vi "centroid detection loop.vi"(7 "CCDs":string[](array[string]), 8 "error in (no error)":errorcluster, 9 "active cams":string[](array[string]), 10 "Detection in":T6 {"detection para"."Particle filtering"."Measurement Parameter" items=["Center of Mass X", "Center of Mass Y", "First Pixel X", "First Pixel Y", "Bounding Rect Left", "Bounding Rect Top", "Bounding Rect Right", "Bounding Rect Bottom", "Max Feret Diameter Start X", "Max Feret Diameter Start Y", "Max Feret Diameter End X", "Max Feret Diameter End Y", "Max Horiz. Segment Length Left", "Max Horiz. Segment Length Right", "Max Horiz. Segment Length Row", "-", "Bounding Rect Width", "Bounding Rect Height", "Bounding Rect Diagonal", "Perimeter", "Convex Hull Perimeter", "Holes' Perimeter", "Max Feret Diameter", "Equivalent Ellipse Major Axis", "Equivalent Ellipse Minor Axis", "Equivalent Ellipse Minor Axis (Feret)", "Equivalent Rect Long Side", "Equivalent Rect Short Side", "Equivalent Rect Diagonal", "Equivalent Rect Short Side (Feret)", "Average Horiz. Segment Length", "Average Vert. Segment Length", "Hydraulic Radius", "Waddel Disk Diameter", "-", "Area", "Holes' Area", "Particle & Holes' Area", "Convex Hull Area", "Image Area", "-", "Number of Holes", "Number of Horiz. Segments", "Number of Vert. Segments", "-", "Orientation", "Max Feret Diameter Orientation", "-", "% Area/Image Area", "% Area/(Particle & Holes' Area)", "Ratio of Equivalent Ellipse Axes", "Ratio of Equivalent Rect Sides", "-", "Elongation Factor", "Compactness Factor", "Heywood Circularity Factor", "Type Factor", "-", "Sum X", "Sum Y", "Sum XX", "Sum XY", "Sum YY", "Sum XXX", "Sum XXY", "Sum XYY", "Sum YYY", "-", "Moment of Inertia XX", "Moment of Inertia XY", "Moment of Inertia YY", "Moment of Inertia XXX", "Moment of Inertia XXY", "Moment of Inertia XYY", "Moment of Inertia YYY", "Norm. Moment of Inertia XX", "Norm. Moment of Inertia XY", "Norm. Moment of Inertia YY", "Norm. Moment of Inertia XXX", "Norm. Moment of Inertia XXY", "Norm. Moment of Inertia XYY", "Norm. Moment of Inertia YYY", "Hu Moment 1", "Hu Moment 2", "Hu Moment 3", "Hu Moment 4", "Hu Moment 5", "Hu Moment 6", "Hu Moment 7"]; "detection para"."Particle filtering"."Range Lower Value" format="%.2f"; "detection para"."Particle filtering"."Range Upper Value" format="%.2f"; "detection para"."detection method" items=["clustering", "entropy", "metric", "moments", "inter-class variance"]; "detection para"."Filter" items=["No Filter", "Median Filter", "Low Pass Filter"]}, 11 "autodetect":bool) -> (0 "error out":errorcluster, 1 "# where centr y is 0":i32[](array[numeric]), 2 "Detection out":T5 {"detection para"."Particle filtering"."Measurement Parameter" items=["Center of Mass X", "Center of Mass Y", "First Pixel X", "First Pixel Y", "Bounding Rect Left", "Bounding Rect Top", "Bounding Rect Right", "Bounding Rect Bottom", "Max Feret Diameter Start X", "Max Feret Diameter Start Y", "Max Feret Diameter End X", "Max Feret Diameter End Y", "Max Horiz. Segment Length Left", "Max Horiz. Segment Length Right", "Max Horiz. Segment Length Row", "-", "Bounding Rect Width", "Bounding Rect Height", "Bounding Rect Diagonal", "Perimeter", "Convex Hull Perimeter", "Holes' Perimeter", "Max Feret Diameter", "Equivalent Ellipse Major Axis", "Equivalent Ellipse Minor Axis", "Equivalent Ellipse Minor Axis (Feret)", "Equivalent Rect Long Side", "Equivalent Rect Short Side", "Equivalent Rect Diagonal", "Equivalent Rect Short Side (Feret)", "Average Horiz. Segment Length", "Average Vert. Segment Length", "Hydraulic Radius", "Waddel Disk Diameter", "-", "Area", "Holes' Area", "Particle & Holes' Area", "Convex Hull Area", "Image Area", "-", "Number of Holes", "Number of Horiz. Segments", "Number of Vert. Segments", "-", "Orientation", "Max Feret Diameter Orientation", "-", "% Area/Image Area", "% Area/(Particle & Holes' Area)", "Ratio of Equivalent Ellipse Axes", "Ratio of Equivalent Rect Sides", "-", "Elongation Factor", "Compactness Factor", "Heywood Circularity Factor", "Type Factor", "-", "Sum X", "Sum Y", "Sum XX", "Sum XY", "Sum YY", "Sum XXX", "Sum XXY", "Sum XYY", "Sum YYY", "-", "Moment of Inertia XX", "Moment of Inertia XY", "Moment of Inertia YY", "Moment of Inertia XXX", "Moment of Inertia XXY", "Moment of Inertia XYY", "Moment of Inertia YYY", "Norm. Moment of Inertia XX", "Norm. Moment of Inertia XY", "Norm. Moment of Inertia YY", "Norm. Moment of Inertia XXX", "Norm. Moment of Inertia XXY", "Norm. Moment of Inertia XYY", "Norm. Moment of Inertia YYY", "Hu Moment 1", "Hu Moment 2", "Hu Moment 3", "Hu Moment 4", "Hu Moment 5", "Hu Moment 6", "Hu Moment 7"]; "detection para"."Particle filtering"."Range Lower Value" format="%.2f"; "detection para"."Particle filtering"."Range Upper Value" format="%.2f"; "detection para"."detection method" items=["clustering", "entropy", "metric", "moments", "inter-class variance"]; "detection para"."Filter" items=["No Filter", "Median Filter", "Low Pass Filter"]}, 3 "bounding rectangle":T1(array[cluster]), 4 "detected array":bool[](array[boolean]), 5 "Particle Reports (Pixels)":T2(array[cluster]))   [LabVIEW 2020]
uses:
  Ctrs/Detection all.ctl
  Ctrs/beam detection.ctl
  <userlib>/_OpenG.lib/array/array.llb/Filter 1D Array with Scalar (String)__ogtk.vi
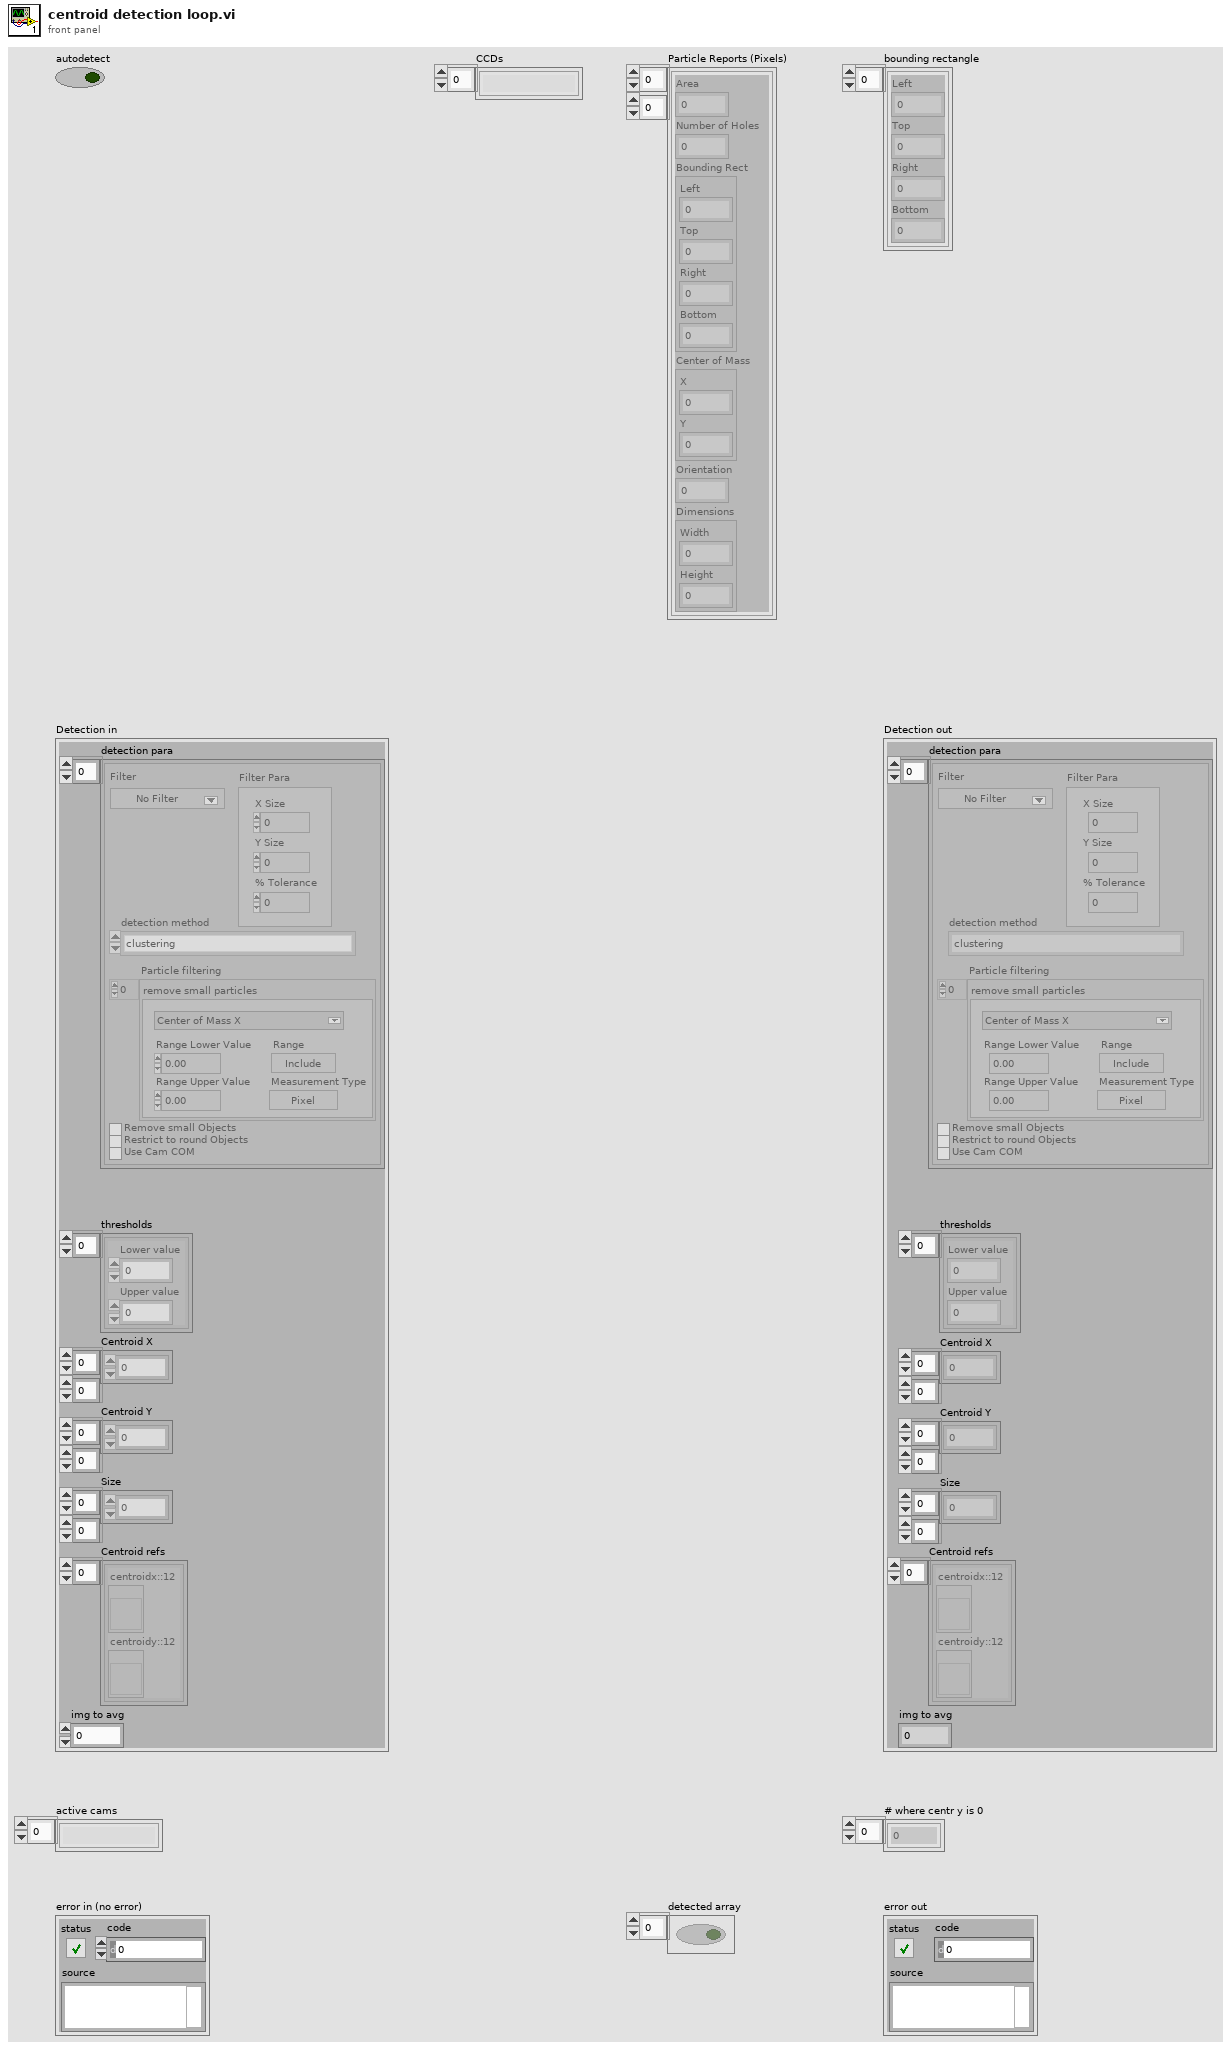
[diagram p1: front panel]
types:
  T1 = cluster{"Left":dbl, "Top":dbl, "Right":dbl, "Bottom":dbl}[]
  T2 = cluster{"Area":dbl, "Number of Holes":dbl, "Bounding Rect":cluster{"Left":dbl, "Top":dbl, "Right":dbl, "Bottom":dbl}, "Center of Mass":cluster{"X":dbl, "Y":dbl}, "Orientation":dbl, "Dimensions":cluster{"Width":dbl, "Height":dbl}}[][]
  T3 = typedef "beam detection.ctl" = cluster{"Filter":u16, "Filter Para":cluster{"X Size":i32, "Y Size":i32, "% Tolerance":i32}, "detection method":i32, "Particle filtering":cluster{"Measurement Parameter":T4, "Range Lower Value":dbl, "Range Upper Value":dbl, "Range":bool, "Measurement Type":bool}[], "Remove small Objects":bool, "Restrict to round Objects":bool, "Use Cam COM":bool}
  T4 = typedef "Particle Parameters" = i32
  T5 = cluster{"detection para":T3[], "thresholds":cluster{"Lower value":sgl, "Upper value":sgl}[], "Centroid X":dbl[][], "Centroid Y":dbl[][], "Size":dbl[][], "Centroid refs":cluster{"centroidx::12":refnum<vi>, "centroidy::12":refnum<vi>}[], "img to avg":i32}
  T6 = typedef "Detection all.ctl" = cluster{"detection para":T3[], "thresholds":cluster{"Lower value":sgl, "Upper value":sgl}[], "Centroid X":dbl[][], "Centroid Y":dbl[][], "Size":dbl[][], "Centroid refs":cluster{"centroidx::12":refnum<vi>, "centroidy::12":refnum<vi>}[], "img to avg":i32}
  T7 = cluster{"centroidx::12":refnum<vi>, "centroidy::12":refnum<vi>}[]
  T8 = cluster{"centroidx::12":refnum<vi>, "centroidy::12":refnum<vi>}
  T9 = cluster{"Left":dbl, "Top":dbl, "Right":dbl, "Bottom":dbl}
  T10 = cluster{"Area":dbl, "Number of Holes":dbl, "Bounding Rect":cluster{"Left":dbl, "Top":dbl, "Right":dbl, "Bottom":dbl}, "Center of Mass":cluster{"X":dbl, "Y":dbl}, "Orientation":dbl, "Dimensions":cluster{"Width":dbl, "Height":dbl}}[]
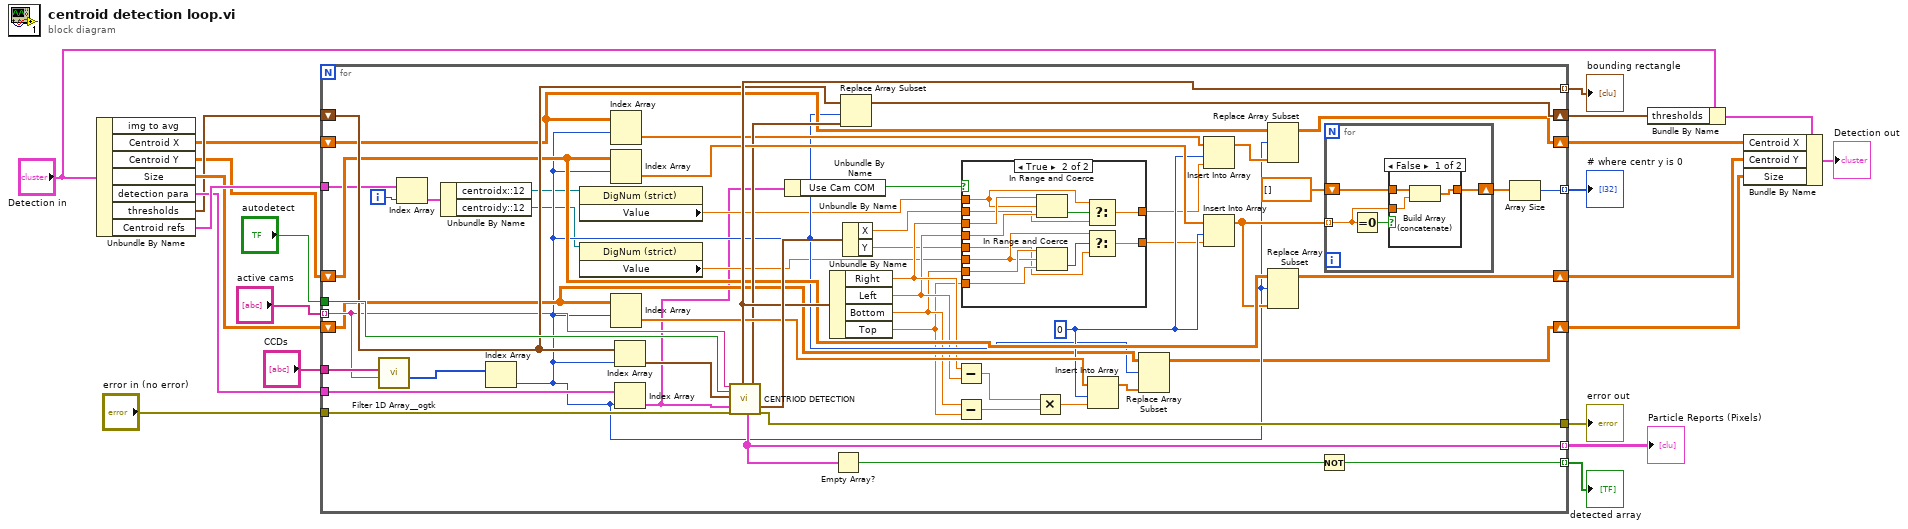
[diagram p0: block diagram]
diagram:
  n1 = Unbundle By Name("Detection in") -> ("Centroid X"=w3:dbl[][], "Centroid Y"=w5:dbl[][], "Size"=w7:dbl[][], "detection para"=w19:T3[], "thresholds"=w6:cluster{"Lower value":sgl, "Upper value":sgl}[], "Centroid refs"=w21:T7)  [unwired: 1 out]
  n2 = for {
    tunnel: "active cams" -> [w54] mode=indexing
    tunnel: [w55] -> w15 mode=indexing
    tunnel: "CCDs" -> [w72]
    tunnel: w19 -> [w70]
    tunnel: [w40] -> w16 mode=indexing
    tunnel: [w68] -> w9 mode=indexing
    tunnel: [w67] -> w2 mode=indexing
    tunnel: "autodetect" -> [w61]
    tunnel: "error in (no error)" -> [w73]
    tunnel: [w74] -> w10
    shift-right: [w58] -> w12
    shift-left: w6 -> [w60]
    shift-right: [w50] -> w18
    shift-left: w3 -> [w52]
    shift-right: [w47] -> w13
    shift-left: w5 -> [w49]
    shift-right: [w41] -> w14
    shift-left: w7 -> [w43]
    tunnel: w21 -> [w39]
    i -> [w38]
    w45 = 0 ("index")
    n3 = call-poly <userlib>:"Filter 1D Array__ogtk.vi"("items to filter"=w54, "array"=w72) -> ("filtered item indices"=w71:i32[])  [unwired: 4 in, 1 out]
    n4 = Index Array(array=w39, index=w38) -> (element=w37:T8)
    n5 = Unbundle By Name(w37) -> ("centroidx::12"=w36:refnum<vi>, "centroidy::12"=w35:refnum<vi>)
    n6 = Index Array(array=w71) -> (element=w42:i32)  [unwired: 1 in]
    n7 = property class="DigNum (strict)"(reference=w36) -> ("Value"=w32:dbl)  [unwired: 1 in, 2 out]
    n8 = property class="DigNum (strict)"(reference=w35) -> ("Value"=w29:dbl)  [unwired: 1 in, 2 out]
    n9 = Index Array(array=w52, index (row)=w42) -> (element=w53:dbl[])  [unwired: 1 in]
    n10 = Index Array(array=w49, index (row)=w42) -> (element=w66:dbl[])  [unwired: 1 in]
    n11 = Index Array(array=w43, index (row)=w42) -> (element=w65:dbl[])  [unwired: 1 in]
    n12 = Index Array(array=w60, index=w42) -> (element=w64:cluster{"Lower value":sgl, "Upper value":sgl})
    n13 = Index Array(array=w70, index=w42) -> (element=w24:T3)
    n14 = call "CENTRIOD DETECTION.vi"("Refnum in"=w54, "auto threshold"=w61, "Threshold Range In"=w64, "beam detection para"=w24, "error in (no error)"=w73) -> ("Bounding Rect"=w67:T9, "Particle Reports (Pixels)"=w68:T10, "Threshold Range Out"=w59:cluster{"Lower value":sgl, "Upper value":sgl}, "Centriod"=w75:cluster{"X":dbl, "Y":dbl}, "error out"=w74:errorcluster)  [unwired: 7 in, 3 out]
    n15 = Unbundle By Name(w24) -> ("Use Cam COM"=w23:bool)
    n16 = Unbundle By Name(w67) -> ("Right"=w34:dbl, "Left"=w33:dbl, "Bottom"=w28:dbl, "Top"=w27:dbl)
    n17 = Empty Array?(array=w68) -> (empty?=w69:bool)
    n18 = Replace Array Subset(array=w60, new element=w59, index=w42) -> (w58:cluster{"Lower value":sgl, "Upper value":sgl}[])
    n19 = Unbundle By Name(w75) -> ("X"=w31:dbl, "Y"=w26:dbl)
    n20 = Subtract(x=w34, y=w33) -> (x-y=w56:dbl)
    n21 = Subtract(x=w28, y=w27) -> (x-y=w57:dbl)
    n22 = case shown="True" w23 {
      tunnel: w34 -> [_ w89]
      tunnel: w33 -> [_ w88]
      tunnel: w32 -> [_ w86]
      tunnel: w31 -> [w77 w85]
      tunnel: [w77 w84] -> w30
      tunnel: w29 -> [_ w80]
      tunnel: w28 -> [_ w83]
      tunnel: w27 -> [_ w82]
      tunnel: w26 -> [w76 w79]
      tunnel: [w76 w78] -> w25
      frame False {
      }
      frame True {
        n23 = In Range and Coerce(upper limit=w89, x=w86, lower limit=w88) -> (In Range?=w87:bool)  [unwired: 1 out]
        n24 = In Range and Coerce(upper limit=w83, x=w80, lower limit=w82) -> (In Range?=w81:bool)  [unwired: 1 out]
        n25 = Select(t=w86, s=w87, f=w85) -> (s? t:f=w84:dbl)
        n26 = Select(t=w80, s=w81, f=w79) -> (s? t:f=w78:dbl)
      }
    }
    n27 = Multiply(x=w56, y=w57) -> (x*y=w46:dbl)
    n28 = Insert Into Array(array=w65, index=w45, new element=w46) -> (w44:dbl[])
    n29 = Replace Array Subset(array=w43, new element=w44, index (row)=w42) -> (w41:dbl[][])  [unwired: 1 in]
    n30 = Insert Into Array(array=w53, index=w45, new element=w30) -> (w51:dbl[])
    n31 = Insert Into Array(array=w66, index=w45, new element=w25) -> (w48:dbl[])
    n32 = Replace Array Subset(array=w52, new element=w51, index (row)=w42) -> (w50:dbl[][])  [unwired: 1 in]
    n33 = Replace Array Subset(array=w49, new element=w48, index (row)=w42) -> (w47:dbl[][])  [unwired: 1 in]
    n34 = Not(x=w69) -> (.not. x?=w40:bool)
    n35 = for {
      shift-right: [w90] -> w62
      shift-left: dbl[] [] ("Array 4") -> [w93]
      tunnel: w48 -> [w91] mode=indexing
      n36 = Equal To 0?(x=w91) -> (x = 0?=w92:bool)
      n37 = case shown="False" w92 {
        tunnel: w93 -> [w96 w97]
        tunnel: w91 -> [w95 _]
        tunnel: [w94 w97] -> w90
        frame False {
          n38 = Build Array (concatenate)(w96, w95) -> (w94:dbl[])
        }
        frame True {
        }
      }
    }
    n39 = Array Size(array=w62) -> (size(s)=w55:i32)
  }
  "detected array" <- w16
  "# where centr y is 0" <- w15
  "error out" <- w10
  "Particle Reports (Pixels)" <- w9
  "bounding rectangle" <- w2
  n40 = Bundle By Name(cluster="Detection in", "thresholds"=w12) -> (w1:T6)
  n41 = Bundle By Name(cluster=w1, "Centroid X"=w18, "Centroid Y"=w13, "Size"=w14) -> (→"Detection out":T6)
